vi "FlushQueue.vi"(8 "error in (no error)":errorcluster, 11 "MessageQueue in":refnum<class "MessageQueue.lvclass">) -> (0 "error out":errorcluster, 2 "Remaining Messages":refnum<class "Message.lvclass">[](array[class]), 3 "MessageQueue out":refnum<class "MessageQueue.lvclass">)   [LabVIEW 2013, in "LapDog.Messaging.v3.lvlib" / "MessageQueue.lvclass"]
doc: "Removes all messages from the queue and returns the messages as an array."
uses:
  MessageQueue.lvclass
  Message/Message.lvclass
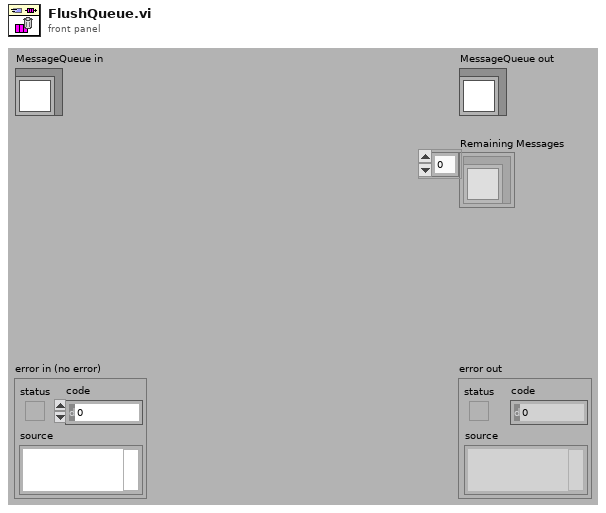
[diagram p1: front panel]
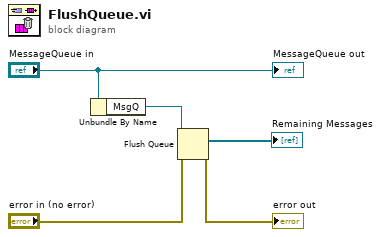
[diagram p0: block diagram]
diagram:
  n1 = Unbundle By Name("MessageQueue in") -> ("MsgQ"=w4:refnum<queue>)
  n2 = Flush Queue(queue=w4, error in (no error)="error in (no error)") -> (remaining elements=→"Remaining Messages":refnum<class "Message.lvclass">[], error out=→"error out":errorcluster)  [unwired: 1 out]
  "MessageQueue out" <- "MessageQueue in"
